vi "Get Right Clicked Object Ref.vi"(8 "error in":errorcluster, 10 "Coords":T1, 11 "Button in":u16) -> (0 "error out":errorcluster, 2 "Button out":u16, 3 "GObject out":refnum<vi>)   [LabVIEW 2012]
uses:
  <vilib>/Utility/miscctls.llb/LVPoint32TypeDef.ctl
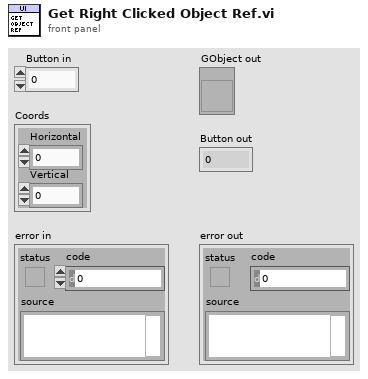
[diagram p1: front panel]
types:
  T1 = typedef "LVPoint32TypeDef.ctl" = cluster{"Horizontal":i32, "Vertical":i32}
  T2 = typedef "LVRectTypeDef.ctl" = cluster{"Left":i16, "Top":i16, "Right":i16, "Bottom":i16}
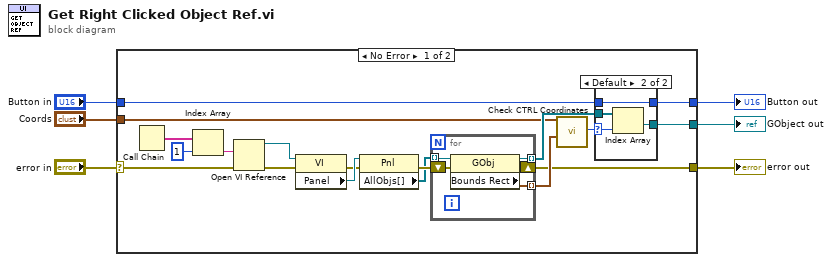
[diagram p0: block diagram]
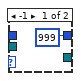
[diagram p2: hidden frame]
diagram:
  n1 = case shown="No Error" "error in" {
    selector: "error in" -> [w8 w35]
    tunnel: [w23 w35] -> w6
    tunnel: [w19 _] -> w5
    tunnel: [w18 _] -> w4
    tunnel: "Button in" -> [w16 _]
    tunnel: "Coords" -> [w15 _]
    frame No Error {
      n2 = Call Chain() -> (call chain=w12:string[])
      n3 = Index Array(array=w12, index=1) -> (element=w10:string)
      n4 = Open VI Reference(vi path=w10, error in (no error)=w8) -> (vi reference=w7:refnum<vi>, error out=w9:errorcluster)  [unwired: 4 in]
      n5 = property class="VI"(reference=w7, error in=w9) -> (error out=w13:errorcluster, "Panel"=w14:refnum<vi>)  [unwired: 1 out]
      n6 = property class="Pnl"(reference=w14, error in=w13) -> (error out=w22:errorcluster, "AllObjs[]"=w20:refnum<vi>[])  [unwired: 1 out]
      n7 = for {
        tunnel: w20 -> [w27] mode=indexing
        tunnel: [w29] -> w24 mode=indexing
        tunnel: [w28] -> w21 mode=indexing
        shift-right: [w25] -> w23
        shift-left: w22 -> [w26]
        n8 = property class="GObj"(reference=w27, error in=w26) -> (reference out=w28:refnum<vi>, error out=w25:errorcluster, "Bounds Rect"=w29:T2)
      }
      n9 = call "Check CTRL Coordinates.vi"("Object Coords Array In"=w24, "Mouse Coords In"=w15) -> ("Index Out"=w17:i32)  [unwired: 9 in]
      n10 = case shown="Default" w17 {
        selector: w17 -> [_ w33]
        tunnel: w21 -> [_ w34]
        tunnel: [_ w32] -> w18
        tunnel: w16 -> [_ w31]
        tunnel: [u16 999 ("Button") w31] -> w19
        frame -1 {
        }
        frame Default {
          n11 = Index Array(array=w34, index=w33) -> (element=w32:refnum<vi>)
        }
      }
    }
    frame Error {
    }
  }
  "error out" <- w6
  "Button out" <- w5
  "GObject out" <- w4
